vi "UE9 eGet DI CR performance tester.vi"() -> (0 "error out":errorcluster)   [LabVIEW 2021]
panel:
  in  "ConnectionType":u16(ring) items=["LJ_ctUSB", "LJ_ctETHERNET"]
  out "Avg ms Per Iteration":dbl format="%.2f"
  out "Total ms":u32
  out "Min Interval":u32
  out "Max Interval":u32
  out "Intervals":u32[](array[numeric])
  in  "Number of Iterations":u32=1000
  in  "stop":bool
  in  "Interval (ms)":u32
  in  "FirstFound":bool=TRUE
  in  "Address":string="192.168.1.209"
  out "Error Message":string
  # "Specify an IP address for Ethernet, or Local ID\nfor USB.  If FirstFound is selected, Local ID is\nignored for USB."
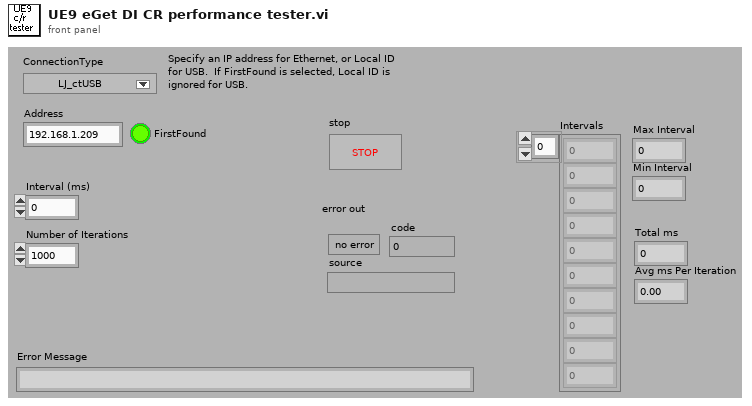
[diagram p1: front panel]
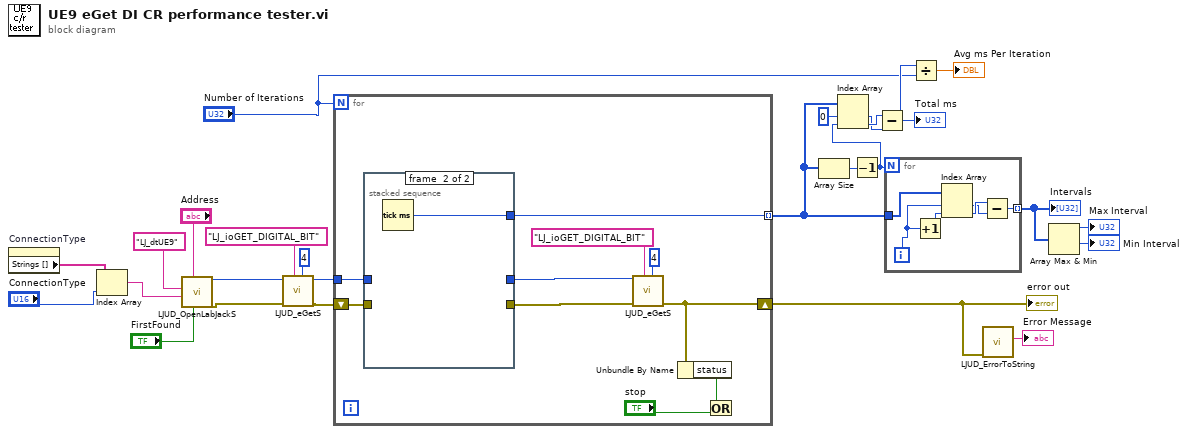
[diagram p0: block diagram]
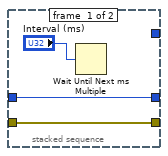
[diagram p2: hidden frame]
diagram:
  n1 = property on="ConnectionType" class="Ring (strict)"() -> ("Strings []"=w9:string[])  [unwired: 2 in, 2 out]
  n2 = Index Array(array=w9, index="ConnectionType") -> (element=w7:string)
  n3 = call "LJUD_OpenLabJackS.vi"("FirstFound"="FirstFound", "Address"="Address", "ConnectionType"=w7, "DeviceType"="LJ_dtUE9") -> ("error out"=w3:errorcluster, "Handle"=w2:i32)  [unwired: 5 in, 1 out]
  n4 = call "LJUD_eGetS.vi"("Channel"=4, "IOType"="LJ_ioGET_DIGITAL_BIT", "error in"=w3, "Handle In"=w2) -> ("error out"=w4:errorcluster, "Handle Out"=w5:i32)  [unwired: 5 in, 1 out]
  n5 = for {
    N: "Number of Iterations" -> [_]
    tunnel: w5 -> [w33]
    shift-right: [w35] -> w22
    shift-left: w4 -> [w32]
    tunnel: [w29] -> w17 mode=indexing
    n6 = stacked-sequence {
      tunnel: w33 -> [w37 _]
      tunnel: w32 -> [w38 _]
      tunnel: [w38 _] -> w31
      tunnel: [w37 _] -> w30
      tunnel: [_ w40] -> w29
      frame #0 {
        n7 = Wait Until Next ms Multiple(millisecond multiple="Interval (ms)") -> ()  [unwired: 1 out]
      }
      frame #1 {
        n8 = Tick Count (ms)() -> (millisecond timer value=w40:u32)
      }
    }
    n9 = call "LJUD_eGetS.vi"("Channel"=4, "IOType"="LJ_ioGET_DIGITAL_BIT", "error in"=w31, "Handle In"=w30) -> ("error out"=w35:errorcluster)  [unwired: 5 in, 2 out]
    n10 = Unbundle By Name(w35) -> ("status"=w36:bool)
    n11 = Or(x=w36, y="stop") -> ()  [unwired: 1 out]
  }
  "error out" <- w22
  n12 = Array Size(array=w17) -> (size(s)=w21:i32)
  n13 = Decrement(x=w21) -> (x-1=w15:i32)
  n14 = Index Array(array=w17, index #1=0 ("Index"), index #2=w15) -> (element #1=w10:u32, element #2=w11:u32)
  n15 = Subtract(x=w11, y=w10) -> (x-y=w14:u32)
  "Total ms" <- w14
  n16 = for {
    N: w15 -> [_]
    tunnel: w17 -> [w46]
    tunnel: [w43] -> w20 mode=indexing
    i -> [w44]
    n17 = Increment(x=w44) -> (x+1=w45:i32)
    n18 = Index Array(array=w46, index #1=w44, index #2=w45) -> (element #1=w41:u32, element #2=w42:u32)
    n19 = Subtract(x=w42, y=w41) -> (x-y=w43:u32)
  }
  "Intervals" <- w20
  n20 = Divide(x=w14, y="Number of Iterations") -> (x/y=→"Avg ms Per Iteration":dbl)
  n21 = call "LJUD_ErrorToString.vi"("error in"=w22) -> ("String"=→"Error Message":string)  [unwired: 10 in]
  n22 = Array Max & Min(array=w20) -> (max value=→"Max Interval":u32, min value=→"Min Interval":u32)  [unwired: 2 out]
